vi "IOScan_StandardizePeriodToMicroSecs.vi"(10 "Units":T1 items=["us", "ms", "secs"], 11 "Period":u32) -> (3 "Period (us)":u32)   [LabVIEW 2016]
uses:
  <resource>/dialog/TargetPreferencePages/IOScan_SubVIs/IOScan_TimeUnit.ctl
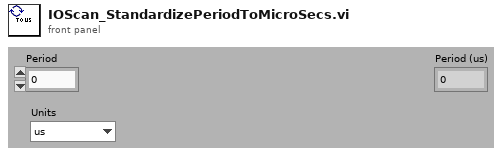
[diagram p1: front panel]
types:
  T1 = typedef "IOScan_TimeUnit.ctl" = u16
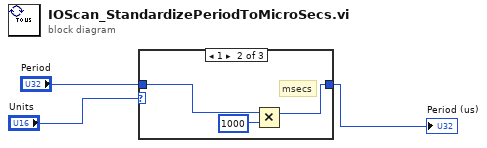
[diagram p0: block diagram]
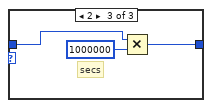
[diagram p3: hidden frame]
diagram:
  n1 = case shown="1" "Units" {
    tunnel: [w4 w5 w8] -> w3
    tunnel: "Period" -> [w4 w7 w10]
    frame 0, Default {
    }
    frame 1 {
      # "msecs"
      n2 = Multiply(x=w7, y=u32 1000) -> (x*y=w5:u32)
    }
    frame 2 {
      # "secs"
      n3 = Multiply(x=w10, y=u32 1000000) -> (x*y=w8:u32)
    }
  }
  "Period (us)" <- w3
